vi "Write SettingsFilename.vi"(8 "error in (no error)":errorcluster, 10 "SettingsFilename":string, 11 "ProgramSettings in":refnum<class "ProgramSettings.lvclass">) -> (0 "error out":errorcluster, 3 "ProgramSettings out":refnum<class "ProgramSettings.lvclass">)   [LabVIEW 2017, in "ProgramSettings.lvclass"]
uses:
  ProgramSettings.lvclass
  ProgramSettings.lvclass/ProgramSettings.ctl
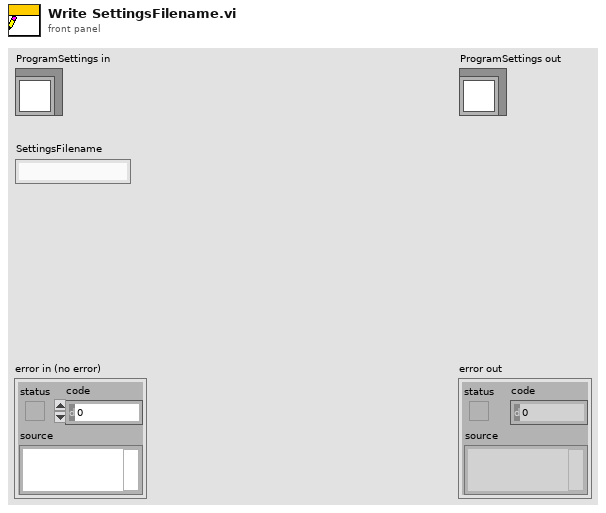
[diagram p1: front panel]
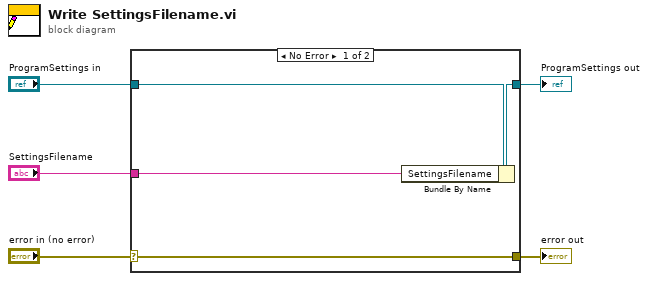
[diagram p0: block diagram]
diagram:
  n1 = case shown="No Error" "error in (no error)" {
    selector: "error in (no error)" -> [w9 w10]
    tunnel: [w9 w10] -> w4
    tunnel: [w7 w11] -> w2
    tunnel: "ProgramSettings in" -> [w8 w11]
    tunnel: "SettingsFilename" -> [w6 _]
    frame No Error {
      n2 = Bundle By Name(cluster=w8, "SettingsFilename"=w6) -> (w7:refnum<class "ProgramSettings.lvclass">)
    }
    frame Error {
    }
  }
  "error out" <- w4
  "ProgramSettings out" <- w2
